vi "RT-HS-Parallel-Port.vi"() -> ()   [LabVIEW 2016]
uses:
  <vilib>/NI/STM/TCP/TCP Connection Info.ctl
  <vilib>/NI/STM/SubVIs/MetaDataElement.ctl
  <vilib>/NI/STM/TCP/Write Meta Data (TCP Ref).vi
  <vilib>/NI/STM/TCP/Read Message (TCP).vi
  <vilib>/FPGAPlugInAG/myRIO-1900/niLvFpga_Open_myRIO-1900.vi
  <vilib>/rvi/interface/common/dynamic/niFpgaDynamicAddResources.vi
  <vilib>/Utility/error.llb/Error Cluster From Error Code.vi
  <vilib>/rvi/errors/niLvFpgaAdjustHostInterfaceError.vi
  <vilib>/rvi/interface/common/niFpgaWaitOnOcc.vi
  <vilib>/FPGAPlugInAG/Dynamic/niLvFpga_Run_Dynamic.vi
  <vilib>/RVI Host/nirviSupport.llb/nirviErrorClusterFromErrorCode.vi
  <vilib>/FPGAPlugInAG/Dynamic/niLvFpga_Abort_Dynamic.vi
  <vilib>/FPGAPlugInAG/Dynamic/niLvFpga_Reset_Dynamic.vi
  <vilib>/FPGAPlugInAG/Dynamic/niLvFpga_Close_Dynamic.vi
  <vilib>/NI/STM/TCP/Write Message (TCP).vi
  <vilib>/NI/STM/TCP/Write Meta Data (TCP Clst).vi
  <vilib>/rvi/interface/nirviOpenFPGA/nirviOpenFPGA.xnode
  FPGA Bitfiles/MyRIO-HS-Paralle_FPGATarget_FPGA-HS-Parallel_x9ODx5NBTEA.lvbitx
  FPGA-HS-Parallel-Port-Receiver.vi
  <vilib>/rvi/interface/nirviReadWriteControl/nirviReadWriteControl.xnode
  <vilib>/rvi/interface/nirviMethod/nirviMethod.xnode
  <vilib>/rvi/interface/nirviCloseFPGA/nirviCloseFPGA.xnode
  <vilib>/rvi/errors/niLvFpgaMergeErrorWithErrorCode.vi
  <vilib>/FPGAPlugInAG/Dynamic/niLvFpga_AcknowledgeIrq_Dynamic.vi
  <vilib>/rvi/interface/nirviMethod/StockFPGA_InlinedMethodWaitForSingleIRQ.vi
  <vilib>/FPGAPlugInAG/Dynamic/niLvFpga_WaitOnIrq_Dynamic.vi
  <vilib>/NI/STM/NI STM.lvlib
  <vilib>/FPGAPlugInAG/Dynamic/niLvFpga_ReadFifo_Dynamic.vi
  <vilib>/rvi/interface/Simulation/niFpgaSimulationCallBeginRW.vi
  NiFpgaLv.dll
  <vilib>/FPGAPlugInAG/Dynamic/niLvFpga_ConfigureFifo_Dynamic.vi
  <vilib>/FPGAPlugInAG/Dynamic/niLvFpga_StartFifo_Dynamic.vi
panel:
  out "CompareVal":u16
  out "OldVal":u16
  out "CurrentIndex":u16
  out "CurrentSample":u16
  in  "StopOnError?":bool
  in  "StepSize":u16=1
  in  "CompArray":u16[](array[numeric])=[0, 1, 2, 3, 4, 5, 6, 7, 8, 9, 10, 11, 12, 13, 14, 15, 16, 17, 18, 19, 20, 21, 22, 23, 24, 25, 26, 27, 28, 29, 30, 31, 32, 33, 34, 35, 36, 37, 38, 39, 40, 41, 42, 43, 44, 45, 46, 47, 48, 49, 50, 51, 52, 53, 54, 55, 56, 57, 58, 59, 60, 61, 62, 63]
  out "Elements Remaining":u32
  in  "Exit":bool
  out "Actual Depth":u32
  out "Data":u32[](array[numeric]) format="%x"
  out "error out":errorcluster
  in  "Timeout (ms)":i32=5000
  in  "#Samples":u32
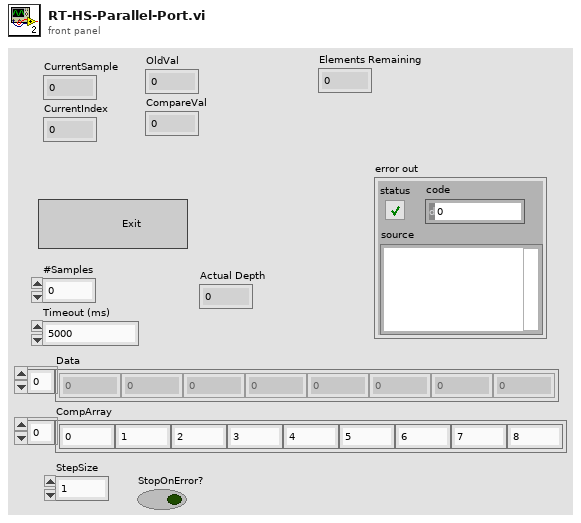
[diagram p1: front panel]
types:
  T1 = typedef "NI STM.lvlib/TCP Connection Info.ctl" = cluster{"connection ID":refnum<k5>, "meta data":T2[]}
  T2 = typedef "NI STM.lvlib/MetaDataElement.ctl" = string
  T3 = enum16{"Read", "Delete", "SetElement", "GetElement", "GetFPelements"}
  T4 = cluster{"Type":string[], "Ref.":refnum<vi>[], "Name":string[]}
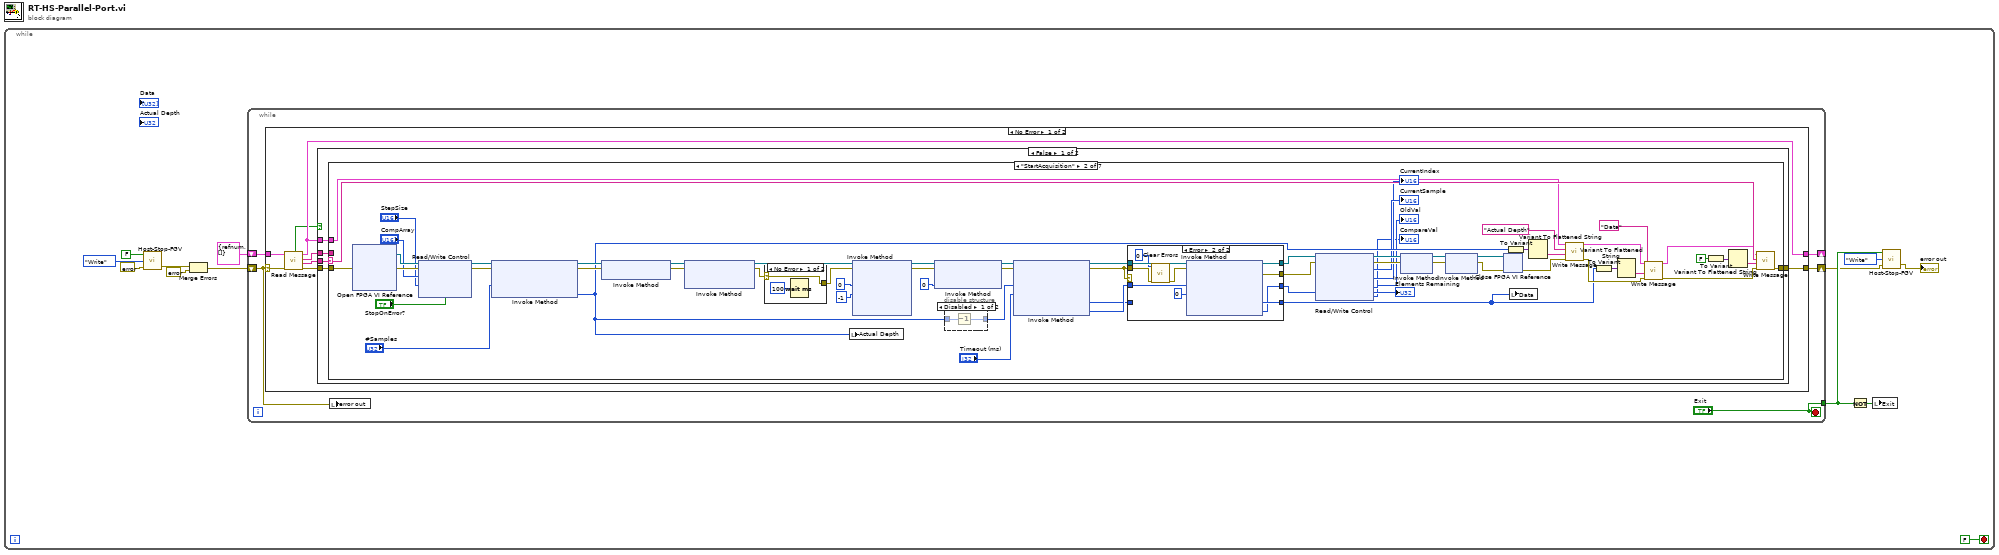
[diagram p0: block diagram]
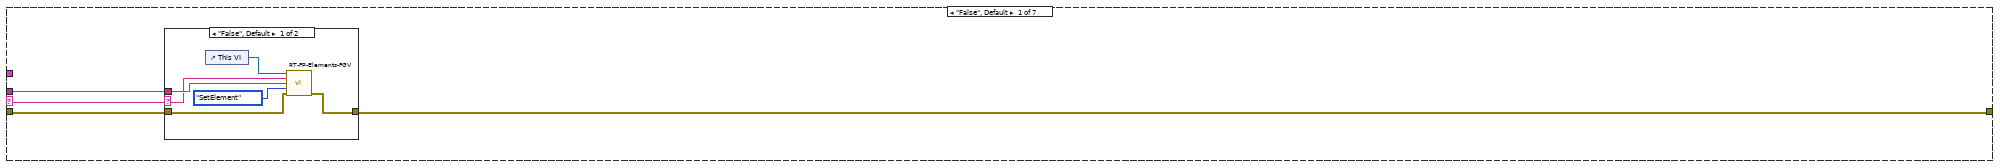
[diagram p2: hidden frame]
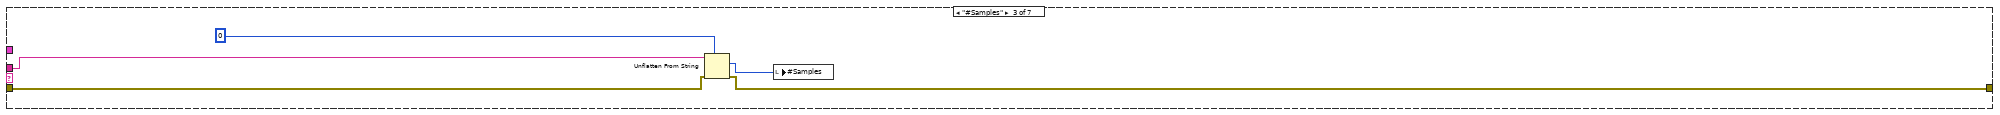
[diagram p7: hidden frame]
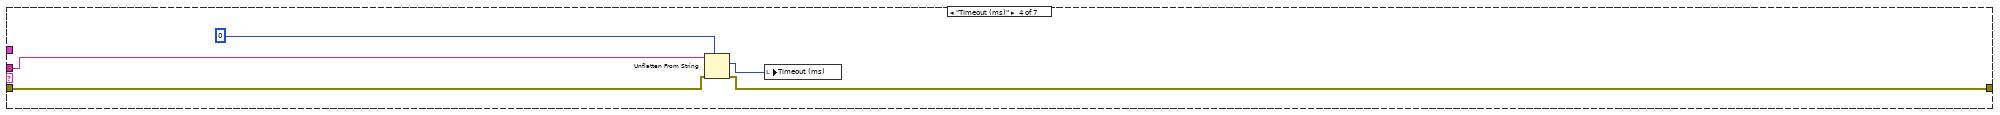
[diagram p8: hidden frame]
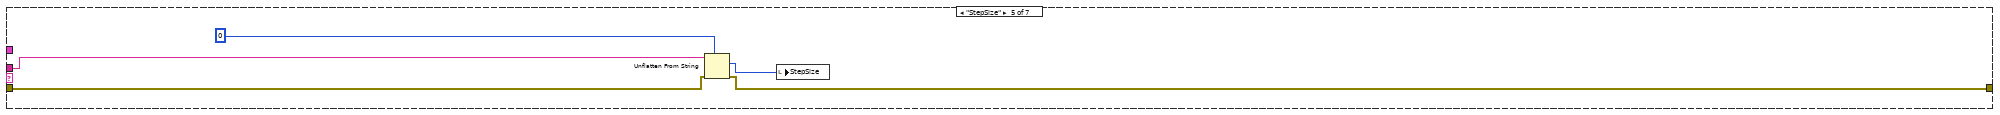
[diagram p9: hidden frame]
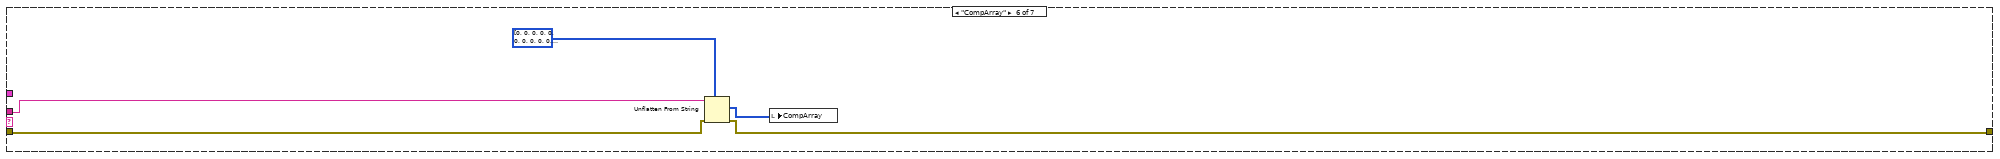
[diagram p10: hidden frame]
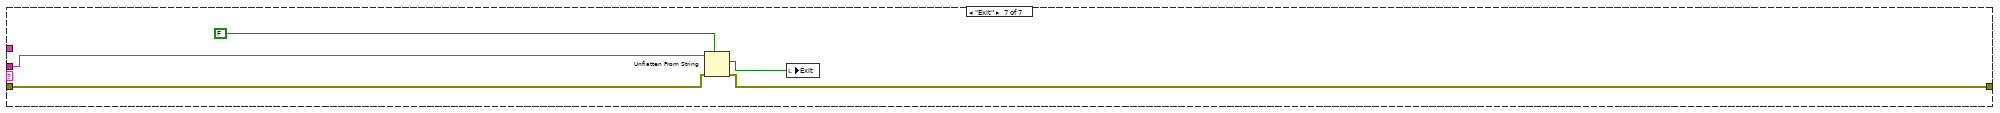
[diagram p11: hidden frame]
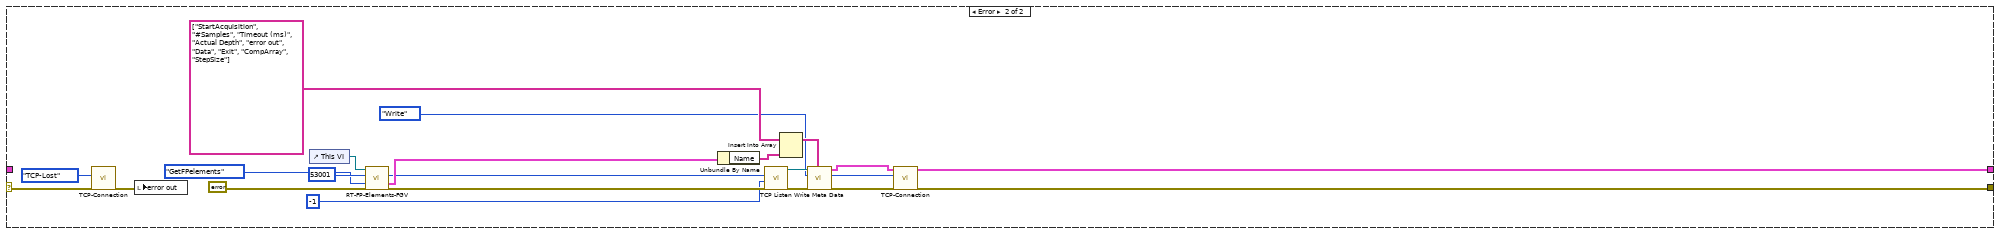
[diagram p13: hidden frame]
diagram:
  n1 = while {
    stop <- FALSE stop-if-true
    n2 = call "Host-Stop-FGV.vi"("error in"=errorcluster {"status"=FALSE, "code"=0, "source"=""}, "Mode"=enum16{"Write", "Read"}."Write", "Stop (in)"=FALSE) -> ("error out"=w12:errorcluster)  [unwired: 1 out]
    n3 = Merge Errors(w12, errorcluster {"status"=TRUE, "code"=0, "source"=""} ("error out")) -> (w2:errorcluster)
    n4 = while {
      shift-right: [w18] -> w5
      shift-left: w2 -> [w14]
      shift-right: [w17] -> _
      shift-left: T1 {"connection ID"=refnum, "meta data"=[]} ("connection info out") -> [w16]
      tunnel: ["Exit"] -> w7
      stop <- "Exit" stop-if-true
      n5 = case shown="No Error" w14 {
        selector: w14 -> [w21 w151]
        tunnel: [w26 w154] -> w18
        tunnel: [w20 w153] -> w17
        tunnel: w16 -> [w22 _]
        frame No Error {
          n6 = call-poly <vilib>:"Read Message.vi"("error in"=w21, "connection info in"=w22) -> ("error out"=w25:errorcluster, "name"=w23:T2, "data string"=w24:string, "connection info out"=w20:T1, "timed out?"=w19:bool)  [unwired: 4 in, 1 out]
          n7 = case shown="False" w19 {
            tunnel: [w31 w149] -> w26
            tunnel: w25 -> [w30 w149]
            tunnel: w24 -> [w29 _]
            tunnel: w23 -> [w28 _]
            tunnel: w20 -> [w27 _]
            frame False {
              n8 = case shown="\"StartAcquisition\"" w28 {
                selector: w28 -> [w32 w99 _ _ _ _ _]
                tunnel: [w33 w100 w124 w129 w134 w141 w144] -> w31
                tunnel: w30 -> [w34 w101 w125 w130 w135 w142 w145]
                tunnel: w29 -> [w35 _ w126 w131 w136 w143 w146]
                tunnel: w27 -> [_ w86 _ _ _ _ _]
                frame "False", Default {
                  n9 = case shown="\"False\", Default" w32 {
                    selector: w32 -> [w36 _]
                    tunnel: w35 -> [w40 _]
                    tunnel: w34 -> [w38 w42]
                    tunnel: [w37 w42] -> w33
                    frame "False", Default {
                      n10 = control-ref of="This VI"() -> (w41:refnum<vi>)
                      n11 = call "RT-FP-Elements-FGV.vi"("VI-ref"=w41, "Name"=w36, "Value in"=w40, "Mode"=T3."SetElement", "error in"=w38) -> ("error out"=w37:errorcluster)  [unwired: 6 in, 4 out]
                    }
                    frame "" {
                    }
                  }
                }
                frame "StartAcquisition" {
                  n12 = xnode "Open FPGA VI Reference"("error in"=w101) -> ("FPGA VI Reference Out"=w56:refnum<k20>, "error out"=w53:errorcluster)  [unwired: 1 in]
                  n13 = xnode "Read/Write Control"("FPGA VI Reference In"=w56, "error in"=w53, "CompArray"="CompArray", "StepSize"="StepSize", "StopOnError?"="StopOnError?") -> ("FPGA VI Reference Out"=w55:refnum<k20>, "error out"=w54:errorcluster)
                  n14 = xnode "Invoke Method"("FPGA VI Reference In"=w55, "error in"=w54, "Requested Depth"="#Samples") -> ("FPGA VI Reference Out"=w68:refnum<k20>, "error out"=w67:errorcluster, "Actual Depth"=w64:u32)
                  n15 = xnode "Invoke Method"("FPGA VI Reference In"=w68, "error in"=w67) -> ("FPGA VI Reference Out"=w66:refnum<k20>, "error out"=w65:errorcluster)
                  n16 = xnode "Invoke Method"("FPGA VI Reference In"=w66, "error in"=w65) -> ("FPGA VI Reference Out"=w69:refnum<k20>, "error out"=w63:errorcluster)  [unwired: 1 in]
                  n17 = case shown="No Error" w63 {
                    selector: w63 -> [w105 w106]
                    tunnel: [w105 w106] -> w62
                    frame No Error {
                      n18 = Wait (ms)(milliseconds to wait=u32 100) -> ()  [unwired: 1 out]
                    }
                    frame Error {
                    }
                  }
                  n19 = local write "Actual Depth"(w64) -> ()
                  n20 = xnode "Invoke Method"("FPGA VI Reference In"=w69, "error in"=w62, "IRQ Number(s)"=0, "Timeout (ms)"=-1) -> ("FPGA VI Reference Out"=w92:refnum<k20>, "error out"=w91:errorcluster)  [unwired: 2 out]
                  n21 = xnode "Invoke Method"("FPGA VI Reference In"=w92, "error in"=w91, "IRQ Number(s)"=0) -> ("FPGA VI Reference Out"=w90:refnum<k20>, "error out"=w89:errorcluster)
                  n22 = disable-structure shown="Disabled" {
                    disable-tunnel: w64 -> [w108 w109]
                    disable-tunnel: [w107 w109] -> w76
                    frame Disabled {
                      n23 = Decrement(x=w108) -> (x-1=w107:u32)
                    }
                    frame Enabled {
                    }
                  }
                  n24 = xnode "Invoke Method"("FPGA VI Reference In"=w90, "error in"=w89, "Number of Elements"=w76, "Timeout (ms)"="Timeout (ms)") -> ("FPGA VI Reference Out"=w74:refnum<k20>, "error out"=w73:errorcluster, "Data"=w71:u32[], "Elements Remaining"=w75:u32)
                  n25 = case shown="Error" w73 {
                    tunnel: w75 -> [w110 w123]
                    tunnel: w73 -> [w112 w116]
                    tunnel: w74 -> [w111 w122]
                    tunnel: [w111 w121] -> w61
                    tunnel: [w112 w120] -> w47
                    tunnel: [w113 w119] -> w72
                    tunnel: w71 -> [w113 _]
                    tunnel: [w110 w117] -> w70
                    frame No Error {
                    }
                    frame Error {
                      n26 = call <vilib>:"Clear Errors.vi"("error in (no error)"=w116, "specific error code to clear (0: all)"=0) -> ("error out"=w115:errorcluster)  [unwired: 4 in, 1 out]
                      n27 = xnode "Invoke Method"("FPGA VI Reference In"=w122, "error in"=w115, "Number of Elements"=w123, "Timeout (ms)"=0) -> ("FPGA VI Reference Out"=w121:refnum<k20>, "error out"=w120:errorcluster, "Data"=w119:u32[], "Elements Remaining"=w117:u32)
                    }
                  }
                  "Elements Remaining" <- w70
                  n28 = xnode "Read/Write Control"("FPGA VI Reference In"=w61, "error in"=w47) -> ("FPGA VI Reference Out"=w49:refnum<k20>, "error out"=w48:errorcluster, "CurrentSample"=→"CurrentSample":u16, "CurrentIndex"=→"CurrentIndex":u16, "OldVal"=→"OldVal":u16, "CompareVal"=→"CompareVal":u16)
                  n29 = xnode "Invoke Method"("FPGA VI Reference In"=w49, "error in"=w48) -> ("FPGA VI Reference Out"=w60:refnum<k20>, "error out"=w59:errorcluster)
                  n30 = xnode "Invoke Method"("FPGA VI Reference In"=w60, "error in"=w59) -> ("FPGA VI Reference Out"=w58:refnum<k20>, "error out"=w57:errorcluster)
                  n31 = xnode "Close FPGA VI Reference"("FPGA VI Reference In"=w58, "error in"=w57) -> ("error out"=w80:errorcluster)
                  n32 = To Variant(anything=w64) -> (Variant=w88:variant)
                  n33 = local write "Data"(w72) -> ()
                  n34 = Variant To Flattened String(Variant=w88) -> (data string=w87:string)  [unwired: 1 out]
                  n35 = call-poly <vilib>:"Write Message.vi"("error in"=w80, "data"=w87, "name"="Actual Depth", "connection info in"=w86) -> ("error out"=w79:errorcluster, "connection info out"=w83:T1)  [unwired: 6 in]
                  n36 = To Variant(anything=w72) -> (Variant=w84:variant)
                  n37 = Variant To Flattened String(Variant=w84) -> (data string=w85:string)  [unwired: 1 out]
                  n38 = call-poly <vilib>:"Write Message.vi"("error in"=w79, "data"=w85, "name"="Data", "connection info in"=w83) -> ("error out"=w77:errorcluster, "connection info out"=w82:T1)  [unwired: 6 in]
                  n39 = To Variant(anything=FALSE) -> (Variant=w96:variant)
                  n40 = Variant To Flattened String(Variant=w96) -> (data string=w98:string)  [unwired: 1 out]
                  n41 = call-poly <vilib>:"Write Message.vi"("error in"=w77, "data"=w98, "name"=w99, "connection info in"=w82) -> ("error out"=w100:errorcluster)  [unwired: 6 in, 1 out]
                }
                frame "#Samples" {
                  n42 = Unflatten From String(type=u32 0, binary string=w126, error in (no error)=w125) -> (value=w128:u32, error out=w124:errorcluster)  [unwired: 2 in, 1 out]
                  n43 = local write "#Samples"(w128) -> ()
                }
                frame "Timeout (ms)" {
                  n44 = Unflatten From String(type=0, binary string=w131, error in (no error)=w130) -> (value=w133:i32, error out=w129:errorcluster)  [unwired: 2 in, 1 out]
                  n45 = local write "Timeout (ms)"(w133) -> ()
                }
                frame "StepSize" {
                  n46 = Unflatten From String(type=u16 0, binary string=w136, error in (no error)=w135) -> (value=w138:u16, error out=w134:errorcluster)  [unwired: 2 in, 1 out]
                  n47 = local write "StepSize"(w138) -> ()
                }
                frame "CompArray" {
                  n48 = Unflatten From String(type=u16[] [0, 0, 0, 0, 0, 0, 0, 0, 0, 0, 0, 0, 0, 0, 0, 0, 0, 0, 0, 0, 0, 0, 0, 0, 0, 0, 0, 0, 0, 0, 0, 0, 0, 0, 0, 0, 0, 0, 0, 0, 0, 0, 0, 0, 0, 0, 0, 0, 0, 0, 0, 0, 0, 0, 0, 0, 0, 0, 0, 0, 0, 0, 0, 0] ("CompArray"), binary string=w143, error in (no error)=w142) -> (value=w139:u16[], error out=w141:errorcluster)  [unwired: 2 in, 1 out]
                  n49 = local write "CompArray"(w139) -> ()
                }
                frame "Exit" {
                  n50 = Unflatten From String(type=FALSE, binary string=w146, error in (no error)=w145) -> (value=w148:bool, error out=w144:errorcluster)  [unwired: 2 in, 1 out]
                  n51 = local write "Exit"(w148) -> ()
                }
              }
            }
            frame True {
            }
          }
        }
        frame Error {
          n52 = call "TCP-Connection.vi"("error in"=w151, "Mode"=enum16{"TCP-Lost", "Write", "Read"}."TCP-Lost") -> ("error out"=w150:errorcluster)  [unwired: 7 in, 2 out]
          n53 = local write "error out"(w150) -> ()
          n54 = control-ref of="This VI"() -> (w160:refnum<vi>)
          n55 = call "RT-FP-Elements-FGV.vi"("VI-ref"=w160, "Mode"=T3."GetFPelements", "error in"=errorcluster {"status"=FALSE, "code"=0, "source"=""} ("error out")) -> ("Cluster"=w164:T4, "error out"=w168:errorcluster)  [unwired: 8 in, 3 out]
          n56 = Unbundle By Name(w164) -> ("Name"=w166:string[])
          n57 = call <vilib>:"TCP Listen.vi"("error in (no error)"=w168, "timeout ms (wait forever: -1)"=-1, "port"=u16 53001) -> ("error out"=w163:errorcluster, "connection ID"=w162:refnum<k5>)  [unwired: 4 in, 3 out]
          n58 = Insert Into Array(array=T2[] ["StartAcquisition", "#Samples", "Timeout (ms)", "Actual Depth", "error out", "Data", "Exit", "CompArray", "StepSize"] ("meta data"), new element=w166) -> (w167:T2[])  [unwired: 1 in]
          n59 = call-poly <vilib>:"Write Meta Data.vi"("meta data"=w167, "error in"=w163, "connection ID"=w162) -> ("error out"=w155:errorcluster, "connection info out"=w156:T1)  [unwired: 7 in]
          n60 = call "TCP-Connection.vi"("error in"=w155, "Mode"=enum16{"TCP-Lost", "Write", "Read"}."Write", "connection info"=w156) -> ("error out"=w154:errorcluster, "connection info Out"=w153:T1)  [unwired: 6 in, 1 out]
        }
      }
      n61 = local write "error out"(w14) -> ()
    }
    n62 = Not(x=w7) -> (.not. x?=w13:bool)
    n63 = local write "Exit"(w13) -> ()
    n64 = call "Host-Stop-FGV.vi"("error in"=w5, "Mode"=enum16{"Write", "Read"}."Write", "Stop (in)"=w7) -> ("error out"=→"error out":errorcluster)  [unwired: 1 out]
  }
